vi "setup_mulit.vi"() -> ()   [LabVIEW 2023]
uses:
  <vilib>/Utility/config.llb/Write Key (Double).vi
  <vilib>/Utility/config.llb/NI_LVConfig.lvlib
panel:
  out "error out 4":errorcluster
  out "max pos":dbl
  out "min pos":dbl
  out "error out 3":errorcluster
  out "error out 2":errorcluster
  out "error out":errorcluster
  in  "stop":bool
  in  "Set zero":bool
  out "position":dbl
  in  "motor ID":i32
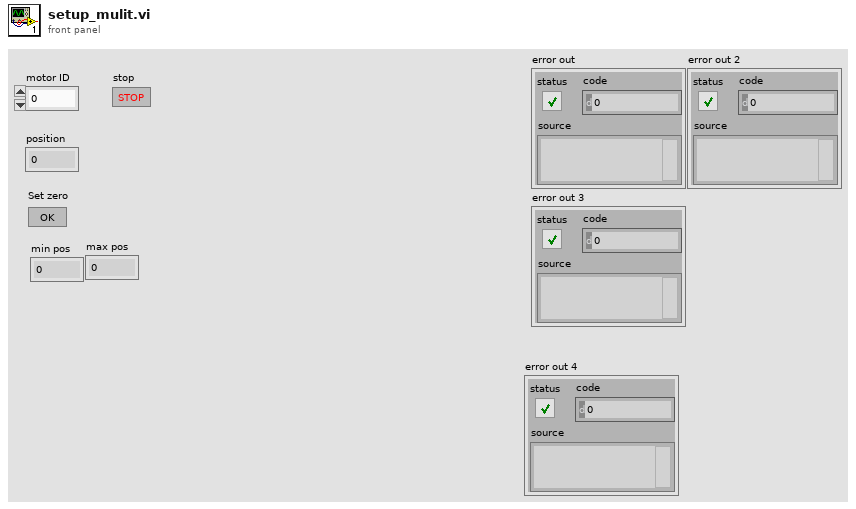
[diagram p1: front panel]
types:
  T1 = typedef "NI_LVConfig.lvlib/Config Data RefNum.ctl" = refnum<k1>
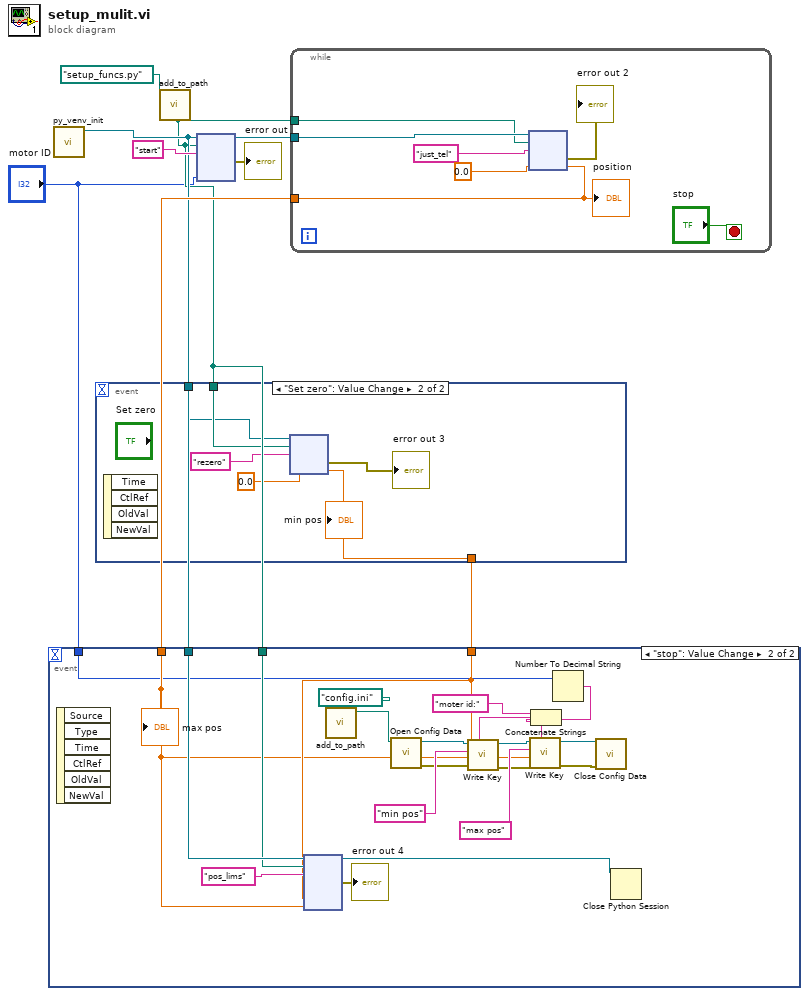
[diagram p0: block diagram]
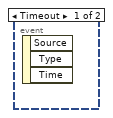
[diagram p2: hidden frame]
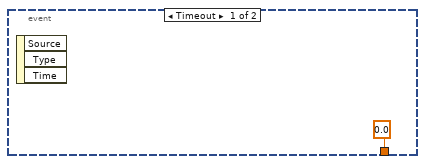
[diagram p3: hidden frame]
diagram:
  n1 = call "py_venv_init.vi"() -> ("Refnum out"=w3:refnum<k35>)  [unwired: 11 in]
  n2 = call "add_to_path.vi"("Path"=path "setup_funcs.py") -> ("appended path"=w2:path)  [unwired: 10 in]
  n3 = event shown="[1] \"Set zero\": Value Change" {
    selector: _ -> [_ _]
    dyn-events: _ -> [_ _]
    timeout: _ -> [_ _]
    tunnel: w3 -> [_ w11]
    tunnel: w2 -> [_ w16]
    tunnel: [0.0 w12] -> w4
    event Timeout {
      n4 = event-data() -> ()  [unwired: 1 in, 3 out]
    }
    event "Set zero": Value Change {
      n5 = event-data() -> ()  [unwired: 1 in, 4 out]
      n6 = node(w11, w16, "rezero" ("function name"), 0.0) -> (→"error out 3":errorcluster, w12:dbl)  [unwired: 1 in, 3 out]
      "min pos" <- w12
    }
  }
  n7 = node(w3, w2, "start", "motor ID") -> (w7:refnum<k35>, →"error out":errorcluster)  [unwired: 4 in, 2 out]
  n8 = while {
    tunnel: w7 -> [w23]
    tunnel: w2 -> [w22]
    tunnel: [w17] -> w5
    stop <- "stop" stop-if-true
    n9 = node(w23, w22, "just_tel", 0.0) -> (→"error out 2":errorcluster, w17:dbl)  [unwired: 1 in, 3 out]
    "position" <- w17
  }
  n10 = event shown="[1] \"stop\": Value Change" {
    selector: _ -> [_ _]
    dyn-events: _ -> [_ _]
    timeout: _ -> [_ _]
    tunnel: w5 -> [_ w30]
    tunnel: w4 -> [_ w31]
    tunnel: w3 -> [_ w34]
    tunnel: w2 -> [_ w33]
    tunnel: "motor ID" -> [_ w27]
    event Timeout {
      n11 = event-data() -> ()  [unwired: 1 in, 3 out]
    }
    event "stop": Value Change {
      n12 = event-data() -> ()  [unwired: 1 in, 6 out]
      n13 = node(w34, w33, "pos_lims" ("function name"), w31, w30) -> (w29:refnum<k35>, →"error out 4":errorcluster)  [unwired: 5 in, 2 out]
      n14 = call "add_to_path.vi"("Path"=path "config.ini") -> ("appended path"=w43:path)  [unwired: 10 in]
      n15 = call <vilib>:"Open Config Data.vi"("configuration file path"=w43) -> ("error out"=w37:errorcluster, "refnum"=w42:T1)  [unwired: 8 in, 1 out]
      n16 = Number To Decimal String(number=w27) -> (decimal integer string=w25:string)  [unwired: 1 in]
      n17 = Concatenate Strings("moter id:", w25) -> (w24:string)
      n18 = call-poly <vilib>:"Write Key.vi"("section"=w24, "error in (no error)"=w37, "value"=w31, "key"="min pos", "refnum"=w42) -> ("error out"=w36:errorcluster, "refnum out"=w40:T1)  [unwired: 4 in, 1 out]
      n19 = call-poly <vilib>:"Write Key.vi"("section"=w24, "error in (no error)"=w36, "value"=w30, "key"="max pos", "refnum"=w40) -> ("error out"=w35:errorcluster, "refnum out"=w38:T1)  [unwired: 4 in, 1 out]
      n20 = call <vilib>:"Close Config Data.vi"("error in (no error)"=w35, "refnum"=w38) -> ()  [unwired: 8 in, 2 out]
      n21 = Close Python Session(session in=w29) -> ()  [unwired: 1 in, 1 out]
      "max pos" <- w30
    }
  }
